vi "Control Motores.vi"(0 "LINX Resource":T2, 1 "Up Button":bool, 2 "Next Button":bool, 5 "Cluster":T1, 7 "Velocidad":dbl(slide) scale=0.0..255.0, 9 "Pause Button":bool, 11 "Error In":errorcluster, 12 "Previous Button":bool, 13 "Down Button":bool) -> (4 "LINX Resource 2":T2, 15 "Error Out":errorcluster)   [LabVIEW 2014]
uses:
  <vilib>/MakerHub/LINX/Private/Type Defs/LINX Ref.ctl
  <vilib>/MakerHub/LINX/Private/Type Defs/Platform.ctl
  <vilib>/MakerHub/LINX/Private/Type Defs/Interface.ctl
  <vilib>/MakerHub/LINX/Private/Device/Type Defs/LINX Device Config.ctl
  <vilib>/MakerHub/LINX/Private/Device/Type Defs/TCP Config.ctl
  <vilib>/MakerHub/LINX/Private/Device/Type Defs/Channels.ctl
  Control Motores.ctl
  <vilib>/MakerHub/LINX/LMH-LINX.lvlib
  <vilib>/MakerHub/LINX/Private/Device/Device.lvlib
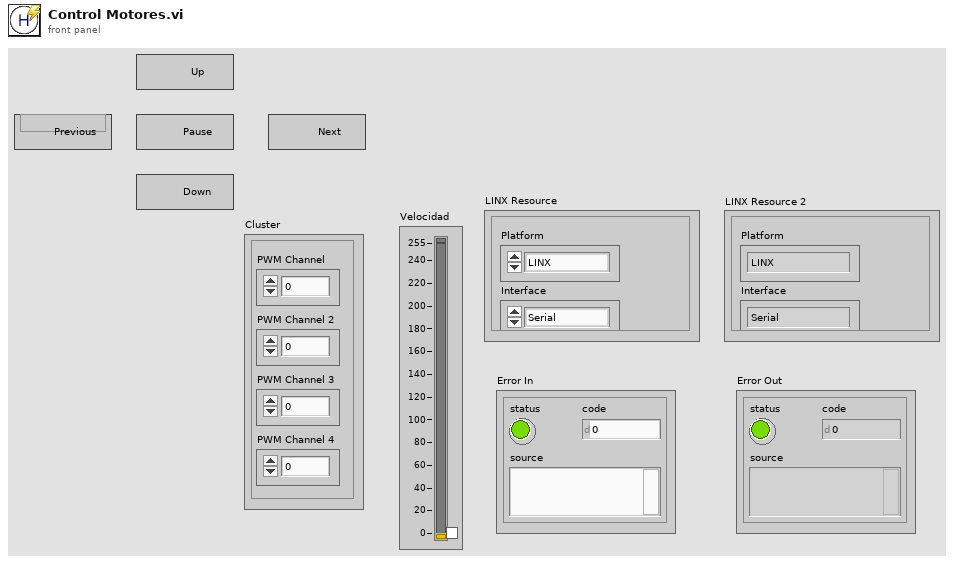
[diagram p1: front panel]
types:
  T1 = cluster{"PWM Channel":u8, "PWM Channel 2":u8, "PWM Channel 3":u8, "PWM Channel 4":u8}
  T2 = typedef "LMH-LINX.lvlib/LINX Ref.ctl" = cluster{"Platform":T3, "Interface":T4, "LINX Device Config":T5}
  T3 = typedef "LMH-LINX.lvlib/Platform.ctl" = enum16{"LINX", "myRIO"}
  T4 = typedef "LMH-LINX.lvlib/Interface.ctl" = enum16{"Serial", "TCP"}
  T5 = typedef "LMH-LINX.lvlib/Device.lvlib/LINX Device Config.ctl" = cluster{"Interface":T4, "COM Port":refnum<visa-resource-name>, "TCP Configuration":T6, "Device Family":u8, "Device ID":u8, "Device Name":string, "TCP Ref":refnum<k5>, "Channels":T7}
  T6 = typedef "LMH-LINX.lvlib/Device.lvlib/TCP Config.ctl" = cluster{"IP Address":string, "Port":u16}
  T7 = typedef "LMH-LINX.lvlib/Channels.ctl" = cluster{"DI":u8[], "DO":u8[], "AI":u8[], "AO":u8[], "PWM":u8[], "QE":u8[], "UART":u8[], "I2C 2":u8[], "SPI":u8[], "CAN":u8[], "Servo":u8[], "AI Ref (V)":dbl, "AO Ref (V)":dbl, "AO Resolution (Bits)":u8}
  T8 = typedef "Control Motores.ctl" = enum16{"Initializer", "Avanza", "Gira Izquierda", "Giro Derecho", "Retrocede", "Pausa"}
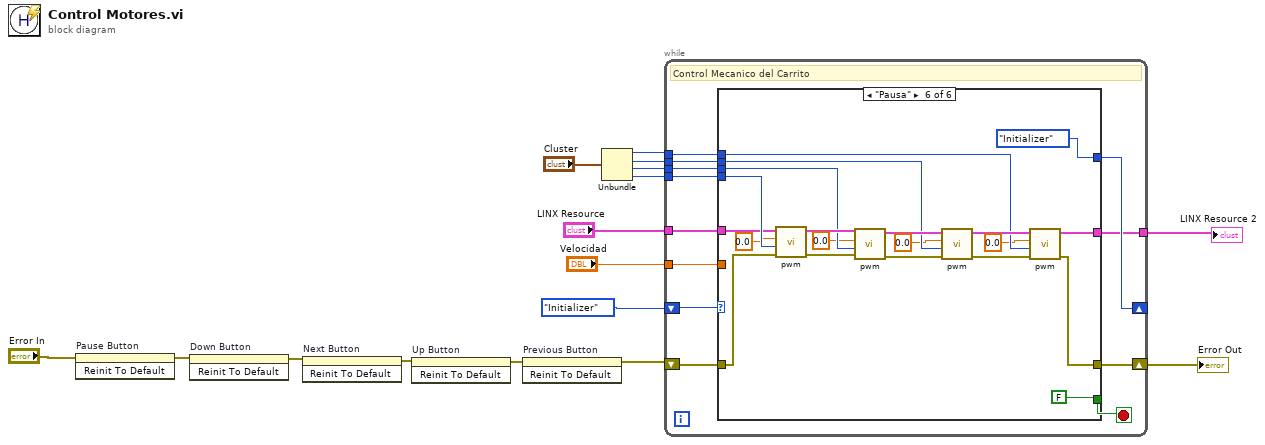
[diagram p0: block diagram]
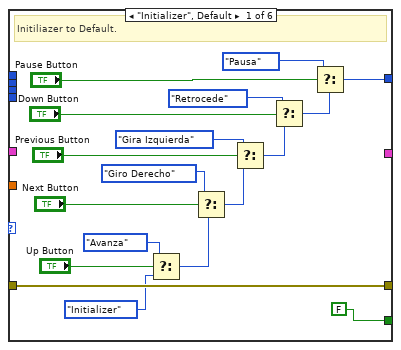
[diagram p2: hidden frame]
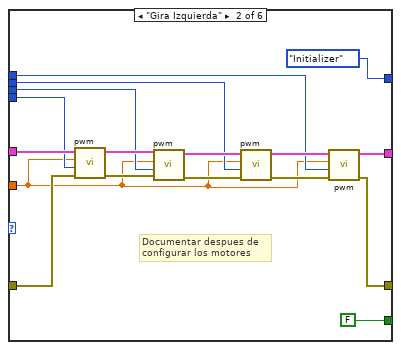
[diagram p3: hidden frame]
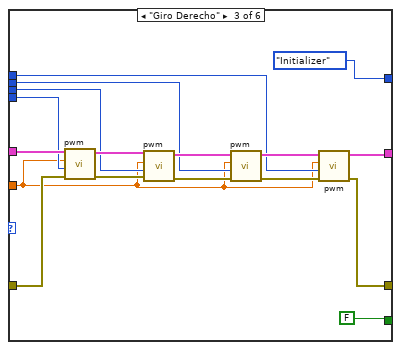
[diagram p4: hidden frame]
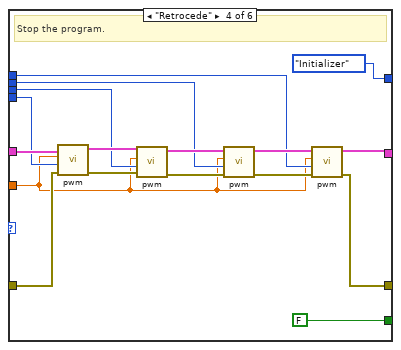
[diagram p5: hidden frame]
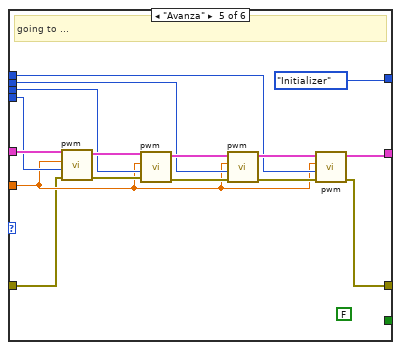
[diagram p6: hidden frame]
diagram:
  n1 = invoke on="Pause Button" class="Bool (strict)" method="Reinit To Default"(error in="Error In") -> (error out=w9:errorcluster)  [unwired: 2 in, 2 out]
  n2 = invoke on="Down Button" class="Bool" method="Reinit To Default"(error in=w9) -> (error out=w10:errorcluster)  [unwired: 2 in, 2 out]
  n3 = invoke on="Next Button" class="Bool" method="Reinit To Default"(error in=w10) -> (error out=w11:errorcluster)  [unwired: 2 in, 2 out]
  n4 = invoke on="Up Button" class="Bool" method="Reinit To Default"(error in=w11) -> (error out=w12:errorcluster)  [unwired: 2 in, 2 out]
  n5 = invoke on="Previous Button" class="Bool" method="Reinit To Default"(error in=w12) -> (error out=w13:errorcluster)  [unwired: 2 in, 2 out]
  n6 = Unbundle("Cluster") -> ("PWM Channel"=w5:u8, "PWM Channel 2"=w4:u8, "PWM Channel 3"=w3:u8, "PWM Channel 4"=w2:u8)
  n7 = while {
    shift-right: [w26] -> _
    shift-left: Control_Motores."Initializer" -> [w17]
    shift-right: [w28] -> w7
    shift-left: w13 -> [w18]
    tunnel: "LINX Resource" -> [w25]
    tunnel: w2 -> [w24]
    tunnel: w3 -> [w23]
    tunnel: w4 -> [w22]
    tunnel: w5 -> [w21]
    tunnel: "Velocidad" -> [w20]
    tunnel: [w19] -> w8
    stop <- w27 stop-if-true
    # "Control Mecanico del Carrito"
    n8 = case shown="\"Pausa\"" w17 {
      tunnel: w18 -> [w46 w56 w72 w85 w100 w123]
      tunnel: [w46 w49 w67 w82 w99 w122] -> w28
      tunnel: [FALSE FALSE FALSE FALSE _ FALSE] -> w27
      tunnel: [w31 Control_Motores."Initializer" Control_Motores."Initializer" Control_Motores."Initializer" Control_Motores."Initializer" Control_Motores."Initializer"] -> w26
      tunnel: w25 -> [_ w59 w74 w90 w107 w121]
      tunnel: w24 -> [_ w55 w73 w89 w106 w127]
      tunnel: w23 -> [_ w54 w71 w88 w105 w126]
      tunnel: w22 -> [_ w53 w70 w87 w104 w125]
      tunnel: w21 -> [_ w52 w69 w86 w103 w124]
      tunnel: w20 -> [_ w51 w68 w84 w102 _]
      tunnel: [_ w50 w66 w83 w101 w120] -> w19
      frame "Initializer", Default {
        # "Initiliazer to Default."
        n9 = Select(t=Control_Motores."Avanza", s="Up Button", f=Control_Motores."Initializer") -> (s? t:f=w43:T8)
        n10 = Select(t=Control_Motores."Giro Derecho", s="Next Button", f=w43) -> (s? t:f=w40:T8)
        n11 = Select(t=Control_Motores."Gira Izquierda", s="Previous Button", f=w40) -> (s? t:f=w37:T8)
        n12 = Select(t=Control_Motores."Retrocede", s="Down Button", f=w37) -> (s? t:f=w34:T8)
        n13 = Select(t=Control_Motores."Pausa", s="Pause Button", f=w34) -> (s? t:f=w31:T8)
      }
      frame "Gira Izquierda" {
        # "Documentar despues de \nconfigurar los motores"
        n14 = call "pwm.vi"("Error In"=w56, "PWM Channel"=w55, "Velocidad"=w51, "LINX Resource"=w59) -> ("Error Out"=w57:errorcluster, "LINX Resource 2"=w58:T2)  [unwired: 6 in]
        n15 = call "pwm.vi"("Error In"=w57, "PWM Channel"=w54, "Velocidad"=w51, "LINX Resource"=w58) -> ("Error Out"=w63:errorcluster, "LINX Resource 2"=w62:T2)  [unwired: 6 in]
        n16 = call "pwm.vi"("Error In"=w63, "PWM Channel"=w53, "Velocidad"=w51, "LINX Resource"=w62) -> ("Error Out"=w61:errorcluster, "LINX Resource 2"=w60:T2)  [unwired: 6 in]
        n17 = call "pwm.vi"("Error In"=w61, "PWM Channel"=w52, "Velocidad"=w51, "LINX Resource"=w60) -> ("Error Out"=w49:errorcluster, "LINX Resource 2"=w50:T2)  [unwired: 6 in]
      }
      frame "Giro Derecho" {
        n18 = call "pwm.vi"("Error In"=w72, "PWM Channel"=w73, "Velocidad"=w68, "LINX Resource"=w74) -> ("Error Out"=w80:errorcluster, "LINX Resource 2"=w79:T2)  [unwired: 6 in]
        n19 = call "pwm.vi"("Error In"=w80, "PWM Channel"=w71, "Velocidad"=w68, "LINX Resource"=w79) -> ("Error Out"=w75:errorcluster, "LINX Resource 2"=w76:T2)  [unwired: 6 in]
        n20 = call "pwm.vi"("Error In"=w75, "PWM Channel"=w70, "Velocidad"=w68, "LINX Resource"=w76) -> ("Error Out"=w77:errorcluster, "LINX Resource 2"=w78:T2)  [unwired: 6 in]
        n21 = call "pwm.vi"("Error In"=w77, "PWM Channel"=w69, "Velocidad"=w68, "LINX Resource"=w78) -> ("Error Out"=w67:errorcluster, "LINX Resource 2"=w66:T2)  [unwired: 6 in]
      }
      frame "Retrocede" {
        # "Stop the program."
        n22 = call "pwm.vi"("Error In"=w85, "PWM Channel"=w89, "Velocidad"=w84, "LINX Resource"=w90) -> ("Error Out"=w96:errorcluster, "LINX Resource 2"=w95:T2)  [unwired: 6 in]
        n23 = call "pwm.vi"("Error In"=w96, "PWM Channel"=w88, "Velocidad"=w84, "LINX Resource"=w95) -> ("Error Out"=w91:errorcluster, "LINX Resource 2"=w92:T2)  [unwired: 6 in]
        n24 = call "pwm.vi"("Error In"=w91, "PWM Channel"=w87, "Velocidad"=w84, "LINX Resource"=w92) -> ("Error Out"=w93:errorcluster, "LINX Resource 2"=w94:T2)  [unwired: 6 in]
        n25 = call "pwm.vi"("Error In"=w93, "PWM Channel"=w86, "Velocidad"=w84, "LINX Resource"=w94) -> ("Error Out"=w82:errorcluster, "LINX Resource 2"=w83:T2)  [unwired: 6 in]
      }
      frame "Avanza" {
        (unwired) FALSE
        # "going to ..."
        n26 = call "pwm.vi"("Error In"=w100, "PWM Channel"=w106, "Velocidad"=w102, "LINX Resource"=w107) -> ("Error Out"=w113:errorcluster, "LINX Resource 2"=w112:T2)  [unwired: 6 in]
        n27 = call "pwm.vi"("Error In"=w113, "PWM Channel"=w105, "Velocidad"=w102, "LINX Resource"=w112) -> ("Error Out"=w108:errorcluster, "LINX Resource 2"=w109:T2)  [unwired: 6 in]
        n28 = call "pwm.vi"("Error In"=w108, "PWM Channel"=w104, "Velocidad"=w102, "LINX Resource"=w109) -> ("Error Out"=w110:errorcluster, "LINX Resource 2"=w111:T2)  [unwired: 6 in]
        n29 = call "pwm.vi"("Error In"=w110, "PWM Channel"=w103, "Velocidad"=w102, "LINX Resource"=w111) -> ("Error Out"=w99:errorcluster, "LINX Resource 2"=w101:T2)  [unwired: 6 in]
      }
      frame "Pausa" {
        n30 = call "pwm.vi"("Error In"=w123, "PWM Channel"=w127, "Velocidad"=0.0, "LINX Resource"=w121) -> ("Error Out"=w128:errorcluster, "LINX Resource 2"=w129:T2)  [unwired: 6 in]
        n31 = call "pwm.vi"("Error In"=w128, "PWM Channel"=w126, "Velocidad"=0.0, "LINX Resource"=w129) -> ("Error Out"=w133:errorcluster, "LINX Resource 2"=w132:T2)  [unwired: 6 in]
        n32 = call "pwm.vi"("Error In"=w133, "PWM Channel"=w125, "Velocidad"=0.0, "LINX Resource"=w132) -> ("Error Out"=w131:errorcluster, "LINX Resource 2"=w130:T2)  [unwired: 6 in]
        n33 = call "pwm.vi"("Error In"=w131, "PWM Channel"=w124, "Velocidad"=0.0, "LINX Resource"=w130) -> ("Error Out"=w122:errorcluster, "LINX Resource 2"=w120:T2)  [unwired: 6 in]
      }
    }
  }
  "LINX Resource 2" <- w8
  "Error Out" <- w7
